vi "Dispose & Terminate.vi"(0 "DBSet in":refnum<class "DBSet.lvclass">, 11 "error in (no error)":errorcluster {"code" format="Error %.0f"}) -> (4 "DBSet out":refnum<class "DBSet.lvclass">, 15 "error out":errorcluster {"code" format="Error %.0f"})   [LabVIEW 2024, in "DBSet.lvclass"]
uses:
  DBSet.lvclass
  DBSet.lvclass/DBSet.ctl
  <vilib>/drjdpowell/SQLite Library/SQL Connection/Connection.lvclass
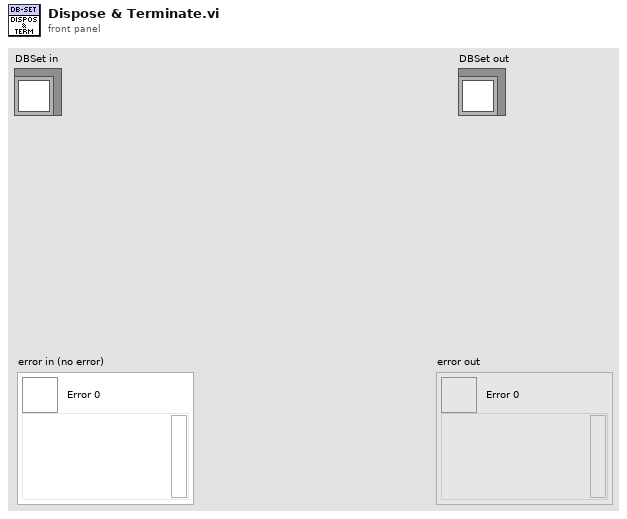
[diagram p1: front panel]
types:
  T1 = typedef "Semaphore RefNum" = refnum<k1>
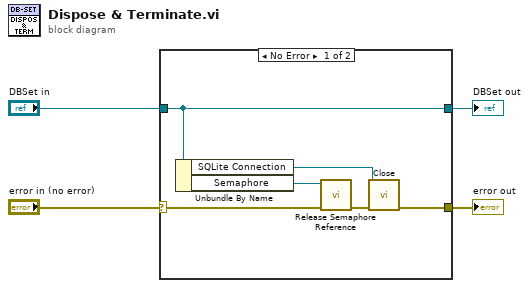
[diagram p0: block diagram]
diagram:
  n1 = case shown="No Error" "error in (no error)" {
    selector: "error in (no error)" -> [w7 w12]
    tunnel: [w5 w12] -> w3
    tunnel: [w6 w11] -> w1
    tunnel: "DBSet in" -> [w6 w11]
    frame No Error {
      n2 = Unbundle By Name(w6) -> ("SQLite Connection"=w10:refnum<class "Connection.lvclass">, "Semaphore"=w8:T1)
      n3 = call <vilib>:"Release Semaphore Reference.vi"("error in (no error)"=w7, "semaphore"=w8) -> ("error out"=w9:errorcluster)  [unwired: 8 in, 1 out]
      n4 = call-dynamic "Close.vi"("error in (no error)"=w9, "SQLite Connection in"=w10) -> ("error out"=w5:errorcluster)  [unwired: 9 in]
    }
    frame Error {
    }
  }
  "error out" <- w3
  "DBSet out" <- w1
